vi "Guitar A440-2.vi"(8 "Frequency":i32, 11 "Samples":i32) -> (3 "Array":dbl[](array[numeric]))   [LabVIEW 2012]
uses:
  <vilib>/ptbypt/NI_PtbyPt.lvlib
panel:
  in  "P":i32(slide) scale=0.0..10.0
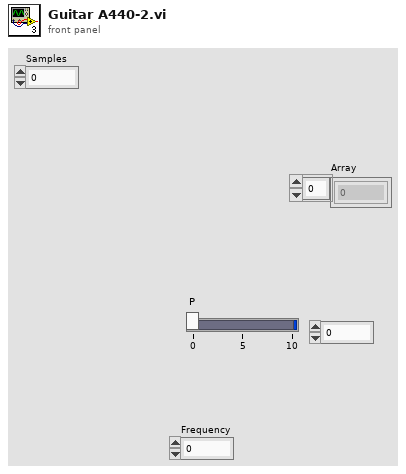
[diagram p1: front panel]
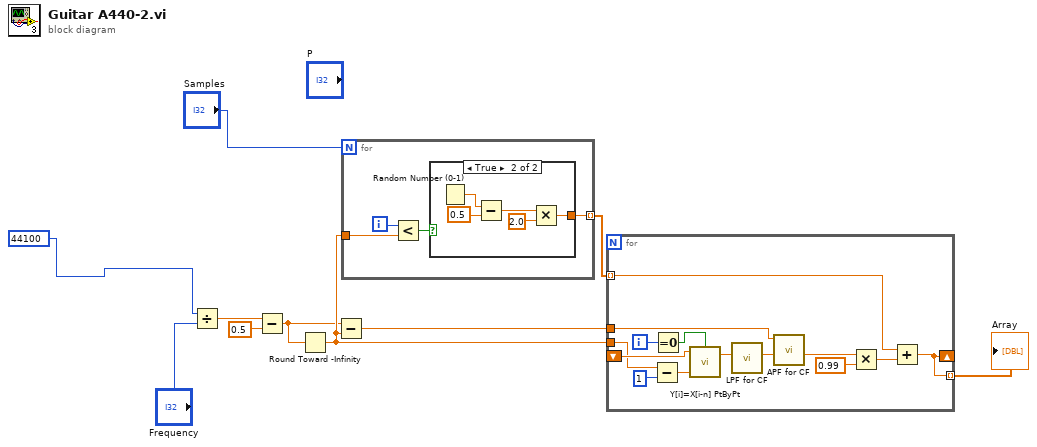
[diagram p0: block diagram]
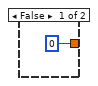
[diagram p2: hidden frame]
diagram:
  n1 = Divide(x=44100, y="Frequency") -> (x/y=w6:dbl)
  n2 = Subtract(x=w6, y=0.5) -> (x-y=w8:dbl)
  n3 = Round Toward -Infinity(1:w8) -> (0:w9:dbl)
  n4 = Subtract(x=w8, y=w9) -> (x-y=w10:dbl)
  n5 = for {
    N: "Samples" -> [_]
    tunnel: [w14] -> w5 mode=indexing
    tunnel: w9 -> [w11]
    i -> [w12]
    n6 = Less?(x=w12, y=w11) -> (x < y?=w13:bool)
    n7 = case shown="True" w13 {
      tunnel: [0 w18] -> w14
      frame False {
      }
      frame True {
        n8 = Random Number (0-1)() -> (number: 0 to 1=w20:dbl)
        n9 = Subtract(x=w20, y=0.5) -> (x-y=w17:dbl)
        n10 = Multiply(x=w17, y=2.0) -> (x*y=w18:dbl)
      }
    }
  }
  n11 = for {
    shift-right: [w29] -> _
    shift-left: _ -> [w31]
    tunnel: [w29] -> w1 mode=indexing
    tunnel: w5 -> [w30] mode=indexing
    tunnel: w9 -> [w28]
    tunnel: w10 -> [w21]
    i -> [w33]
    n12 = Subtract(x=w28, y=1) -> (x-y=w27:dbl)
    n13 = Equal To 0?(x=w33) -> (x = 0?=w32:bool)
    n14 = call <vilib>:"Y[i]=X[i-n] PtByPt.vi"("initialize"=w32, "shifts: n"=w27, "x"=w31) -> ("shifted x"=w25:dbl)  [unwired: 1 in, 1 out]
    n15 = call "LPF for CF.vi"("Numeric"=w25) -> ("Numeric 2"=w23:dbl)  [unwired: 10 in]
    n16 = call "APF for CF.vi"("Input Signal Sample (q)"=w23, "C"=w21) -> ("Output Signal Sample (r)"=w24:dbl)  [unwired: 7 in]
    n17 = Multiply(x=w24, y=0.99) -> (x*y=w34:dbl)
    n18 = Add(x=w30, y=w34) -> (x+y=w29:dbl)
  }
  "Array" <- w1
